vi "Log Status Update.vi"(8 "error in (no error)":errorcluster, 10 "Status":string, 11 "Mag Lab Measure Controller in":refnum<class "Mag Lab Measure Controller.lvclass">) -> (0 "error out":errorcluster, 3 "Mag Lab Measure Controller out":refnum<class "Mag Lab Measure Controller.lvclass">)   [LabVIEW 2015, in "Mag Lab Measure Controller.lvclass"]
uses:
  Mag Lab Measure Controller.lvclass
  Mag Lab Measure Base/Mag Lab Measure Base.lvclass/Mag Lab Measure Base.ctl
  Mag Lab Measure Interface Messages/Log Status Update Msg/Interface Log Status Update Msg.lvclass/Interface Log Status Update Msg.ctl
  <vilib>/ActorFramework/Message Enqueuer/Message Enqueuer.lvclass/Message Enqueuer.ctl
  <vilib>/ActorFramework/Message Enqueuer/Enqueue.vi
  <vilib>/ActorFramework/Message Priority Queue/Priority Enqueue.vi
  <vilib>/ActorFramework/Message Enqueuer/Message Enqueuer.lvclass
  Mag Lab Measure Interface Messages/Log Status Update Msg/Interface Log Status Update Msg.lvclass
  Mag Lab Measure Base/Mag Lab Measure Base.lvclass
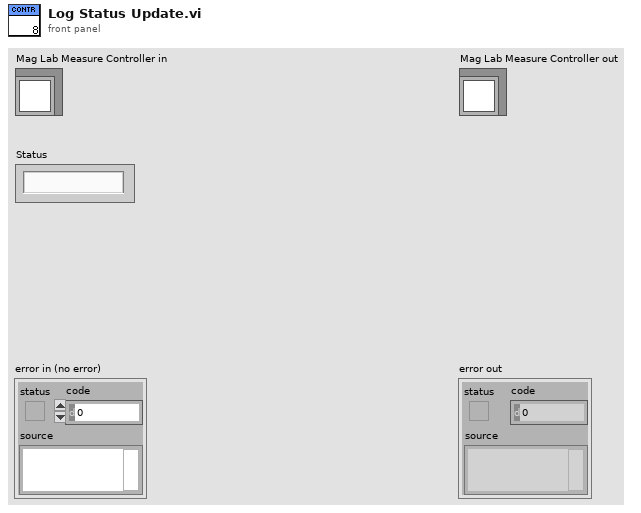
[diagram p1: front panel]
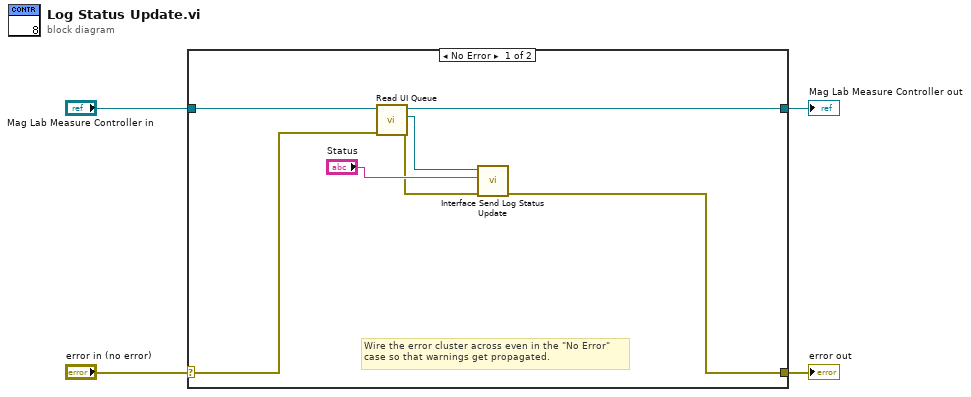
[diagram p0: block diagram]
diagram:
  n1 = case shown="No Error" "error in (no error)" {
    selector: "error in (no error)" -> [w7 w13]
    tunnel: [w5 w13] -> w3
    tunnel: [w11 w12] -> w1
    tunnel: "Mag Lab Measure Controller in" -> [w10 w12]
    frame No Error {
      # "Wire the error cluster across even in the \"No Error\"\ncase so that warnings get propagated."
      n2 = call "Read UI Queue.vi"("error in (no error)"=w7, "Mag Lab Measure Base in"=w10) -> ("error out"=w6:errorcluster, "Actor Framework.lvlib:Message Enqueuer"=w9:refnum<class "Message Enqueuer.lvclass">, "Mag Lab Measure Base out"=w11:refnum<class "Mag Lab Measure Controller.lvclass">)  [unwired: 7 in]
      n3 = call "Interface Send Log Status Update.vi"("error in (no error)"=w6, "Status"="Status", "Message Enqueuer"=w9) -> ("error out"=w5:errorcluster)  [unwired: 7 in, 1 out]
    }
    frame Error {
    }
  }
  "error out" <- w3
  "Mag Lab Measure Controller out" <- w1
